vi "Get Number Of Enum Items.vi"(11 "Enum":variant) -> (3 "Number Of Items":i32)   [LabVIEW 2015, in "Utility.lvlib"]
uses:
  Utility.lvlib
  <vilib>/Utility/Data Type/NI_Data Type.lvlib
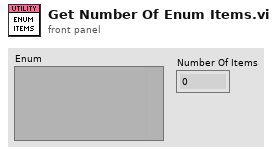
[diagram p1: front panel]
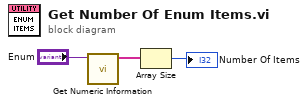
[diagram p0: block diagram]
diagram:
  n1 = call <vilib>:"Get Numeric Information.vi"("Variant"="Enum") -> ("Enum Names"=w2:string[])  [unwired: 7 in, 3 out]
  n2 = Array Size(array=w2) -> (size(s)=→"Number Of Items":i32)
